vi "List file types in folder.vi"(8 "error in (no error)":errorcluster, 11 "Project folder":path) -> (0 "error out":errorcluster, 2 "Binary STAT files":path[](array[path]), 3 "ASCII Logfiles":path[](array[path]))   [LabVIEW 2011]
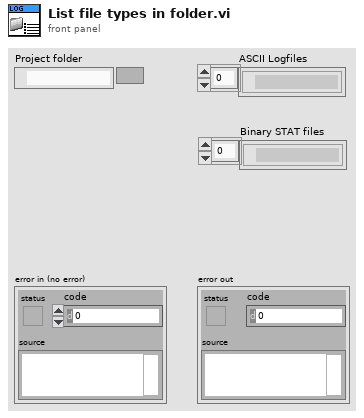
[diagram p1: front panel]
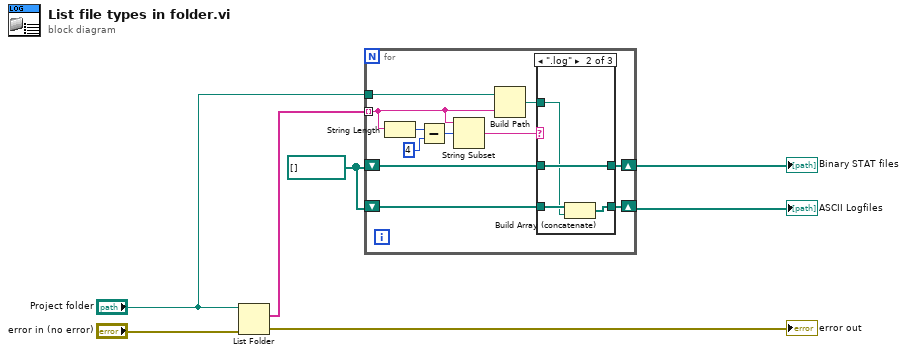
[diagram p0: block diagram]
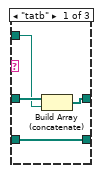
[diagram p2: hidden frame]
diagram:
  w4 = path[] []
  n1 = List Folder(path="Project folder", error in="error in (no error)") -> (filenames=w2:string[], error out=→"error out":errorcluster)  [unwired: 2 in, 2 out]
  n2 = for {
    tunnel: w2 -> [w9] mode=indexing
    shift-right: [w12] -> w1
    shift-left: w4 -> [w14]
    shift-right: [w11] -> w5
    shift-left: w4 -> [w13]
    tunnel: "Project folder" -> [w10]
    n3 = String Length(string=w9) -> (length=w18:i32)
    n4 = Subtract(x=w18, y=4) -> (x-y=w16:i32)
    n5 = String Subset(string=w9, offset (0)=w16) -> (substring=w15:string)  [unwired: 1 in]
    n6 = Build Path(base path=w10, name or relative path=w9) -> (appended path=w8:path)
    n7 = case shown="\".log\"" w15 {
      tunnel: w14 -> [w22 w24 w28]
      tunnel: w13 -> [w20 w26 w27]
      tunnel: [w21 w24 w28] -> w12
      tunnel: [w20 w25 w27] -> w11
      tunnel: w8 -> [w19 w23 _]
      frame "tatb" {
        n8 = Build Array (concatenate)(w22, w19) -> (w21:path[])
      }
      frame ".log" {
        n9 = Build Array (concatenate)(w26, w23) -> (w25:path[])
      }
      frame Default {
      }
    }
  }
  "ASCII Logfiles" <- w5
  "Binary STAT files" <- w1
